vi "convertToHtml.vi"(8 "error in (no error)":errorcluster, 10 "HTML File Path":path, 11 "MS-Excel in":refnum<class "MS-Excel.lvclass">) -> (0 "error out":errorcluster, 3 "MS-Excel out":refnum<class "MS-Excel.lvclass">)   [LabVIEW 2017, in "LabVIEW NPOI.lvlib" / "MS-Excel.lvclass"]
uses:
  MS-Excel.lvclass
  C:/Users/Neo/Desktop/Dev_Tools_BR/LabVIEW_NPOI/lib/NPOI 2.1.1/NPOI.OOXML.dll
  lib/NPOI 2.1.1/NPOI.OOXML.dll
  MS-Excel.lvclass/MS-Excel.ctl
  System.Xml
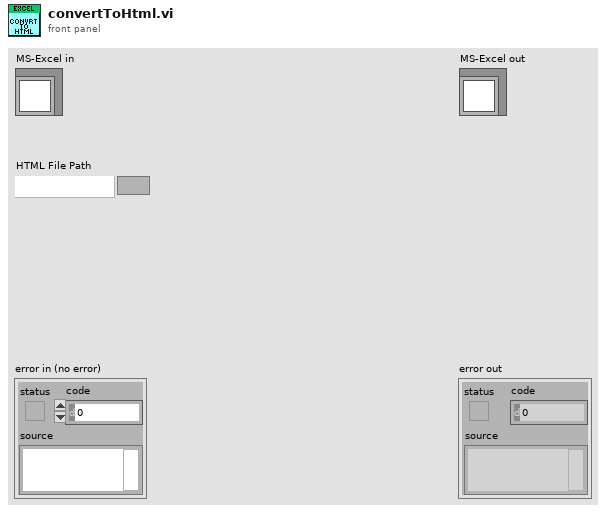
[diagram p1: front panel]
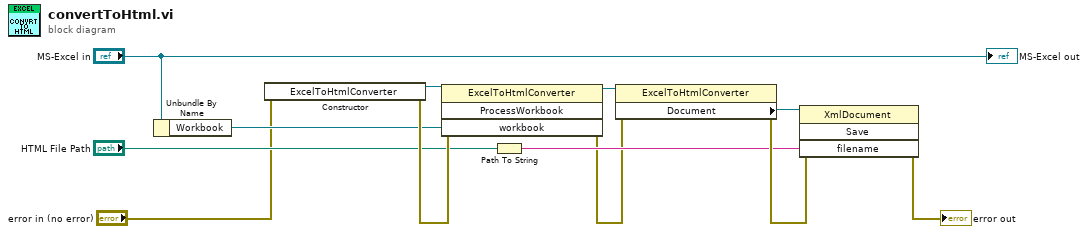
[diagram p0: block diagram]
diagram:
  n1 = Unbundle By Name("MS-Excel in") -> ("Workbook"=w9:refnum<k24>)
  n2 = constructor class="ExcelToHtmlConverter"(error in="error in (no error)") -> (reference out=w11:refnum<k24>, error out=w12:errorcluster)  [unwired: 2 in, 1 out]
  n3 = invoke class="ExcelToHtmlConverter" method="ProcessWorkbook"(reference=w11, error in=w12, "workbook"=w9) -> (reference out=w8:refnum<k24>, error out=w1:errorcluster)  [unwired: 1 in, 2 out]
  n4 = Path To String(path="HTML File Path") -> (string=w4:string)
  n5 = property class="ExcelToHtmlConverter"(reference=w8, error in=w1) -> (error out=w7:errorcluster, "Document"=w6:refnum<k24>)  [unwired: 1 out]
  n6 = invoke class="XmlDocument" method="Save"(reference=w6, error in=w7, "filename"=w4) -> (error out=→"error out":errorcluster)  [unwired: 1 in, 3 out]
  "MS-Excel out" <- "MS-Excel in"
